vi "SystemdBControl.vi"(5 "Command":T1=enum."Connect dB", 6 "error in (no error)":errorcluster={"status"=TRUE, "code"=-2147467259, "source"="Exception occured in Microsoft OLE DB Provider for ODBC Drivers: no such table: sysconfig (1) in ADO Connection Execute.vi->SQL Execute.vi->dBManagerSQLite.vi->SystemdBControl.vi->ConfigSQLite.lvclass:ConfigGetLatestVersion.vi->SQLiteConfigOOP.vi->ConfigSQLiteOOP ini.vi\r\nSQL:Select Distinct\n  sysconfig.idsysconfig\nFrom\n  sysconfig\nOrder By\n  sysconfig.idsysconfig Desc\r\nSQL:Select\n  sysconfig.*\nFrom\n  sysconfig\nWhere\n  sysconfig.idsysconfig =   And\n  sysconfig.SectionName = \"\""}, 9 "Data In":variant) -> (0 "error out":errorcluster, 2 "Empty?":bool, 3 "Data Out":string[][](array[string]))   [LabVIEW 2023]
doc: "*-----------------------------------------------------\n* Author: SWatts\n*\n* VI Description: dB for all config stuff\n* \n*\n* Error handling: All errors passed out\n*\n* Pre-condition: \n*\n* Post-condition: None\n*\n* Revision History:\n*\n* Rev Date Author Description \n* 01 30/04/2014 SWatts First issue\n*\n*-----------------------------------------------------"
uses:
  SQLite/SQLiteLCOD.lvlib
  SQLite/SQLiteLCOD.ctl
  SystemdBCommands.ctl
panel:
  # "Input Data"
  # "Local Data"
  # "Output Data"
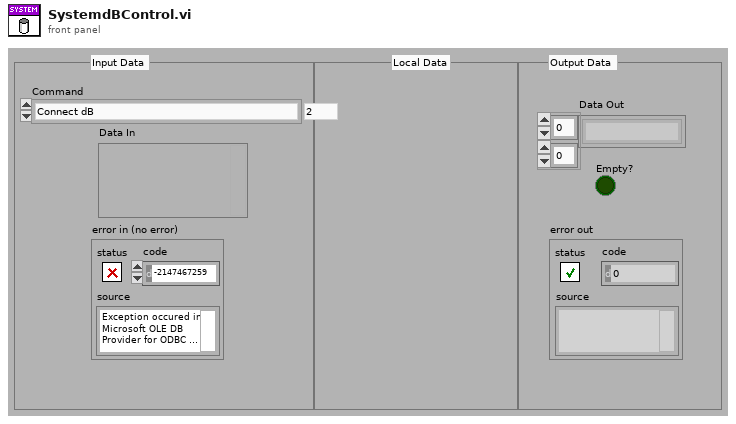
[diagram p1: front panel]
types:
  T1 = typedef "SystemdBCommands.ctl" = enum16{"No Command - Error", "Set Filepath", "Connect dB", "Disconnect dB", "Start Transaction", "Commit", "Rollback", "Describe Table", "Select All From Table", "Fetch Query", "Count Records In Table", "Get User Information", "Get System Config", "Insert New System Config", "UPDATE User Info", "Insert New User", "Get Versions", "Update Key", "Set Version to Default", "Get Default Version", "INSERT Error", "UPDATE Error", "DELETE Errors", "Get All Errors", "Get #Errors for Error"}
  T2 = typedef "SQLiteLCOD.lvlib/SQLiteLCOD.ctl" = enum16{"No Command - Error", "Open", "SQL", "Close", "Prepare SQL", "INSERT Waveform", "INSERT LongText", "Finalise SQL"}
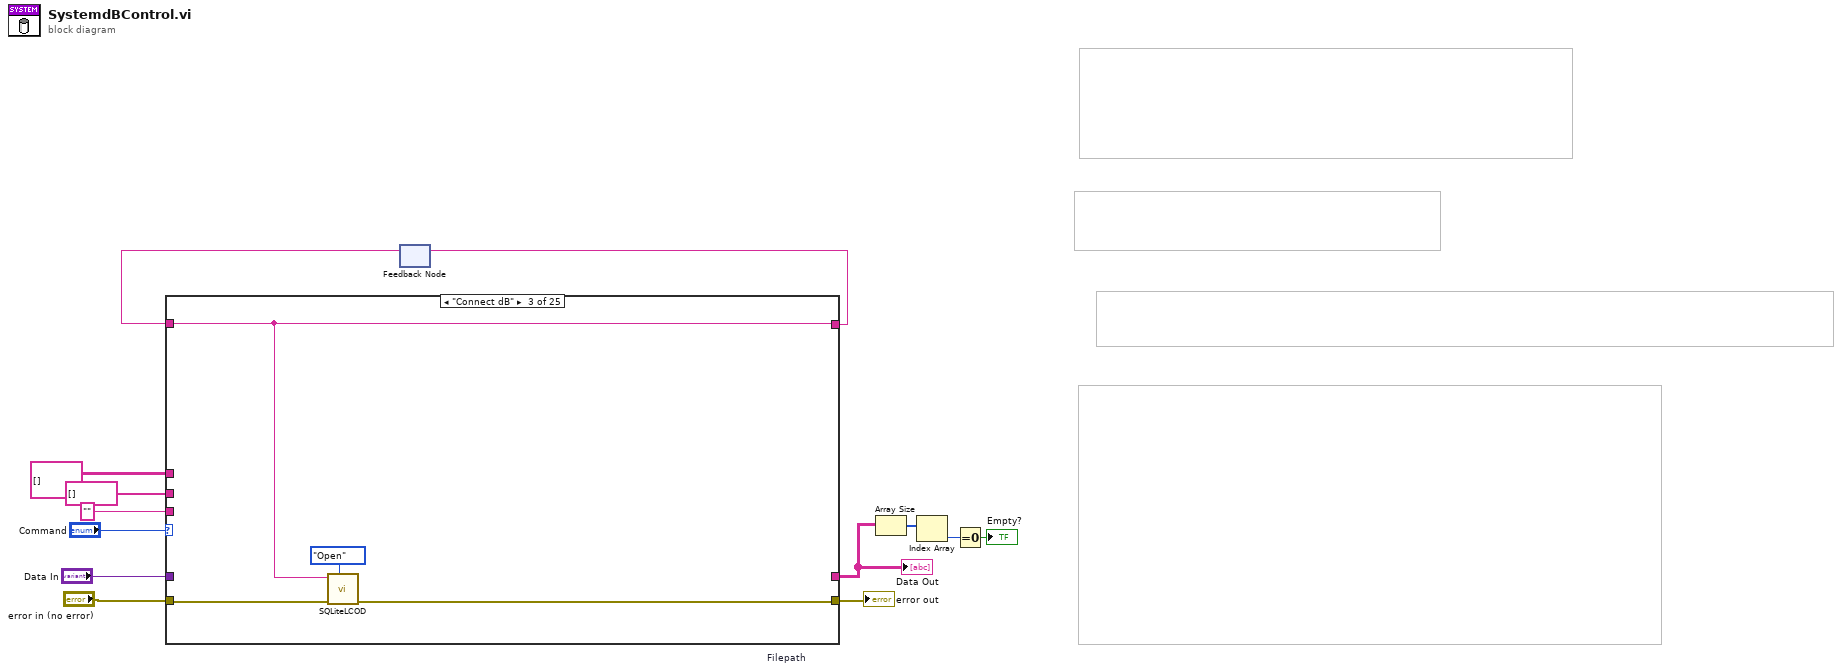
[diagram p0: block diagram]
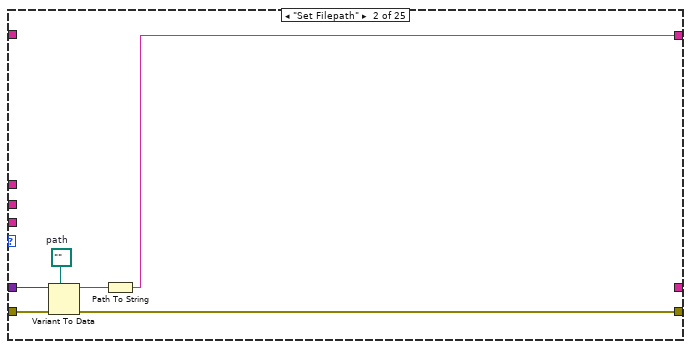
[diagram p3: hidden frame]
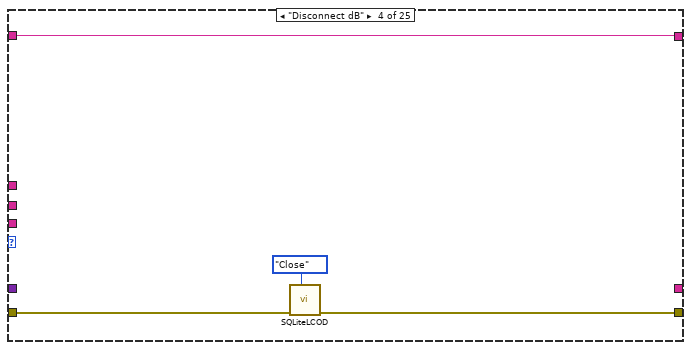
[diagram p4: hidden frame]
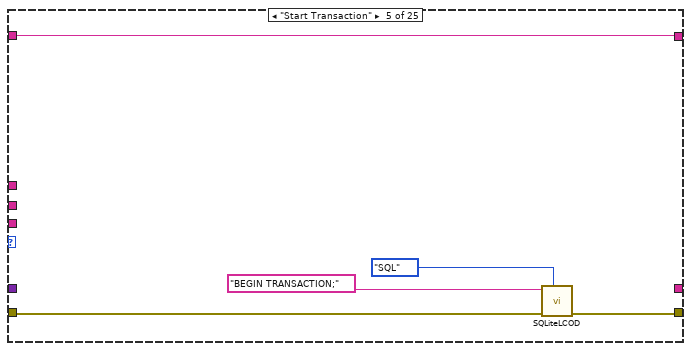
[diagram p5: hidden frame]
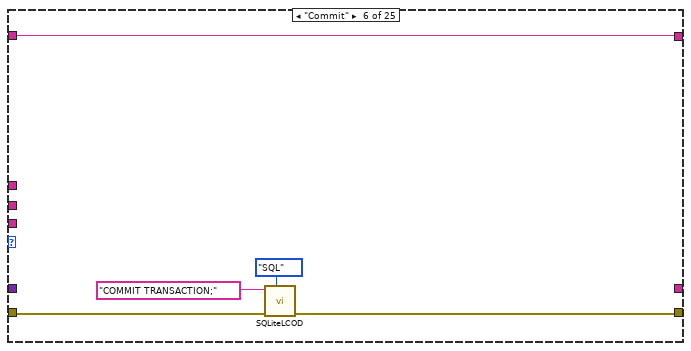
[diagram p6: hidden frame]
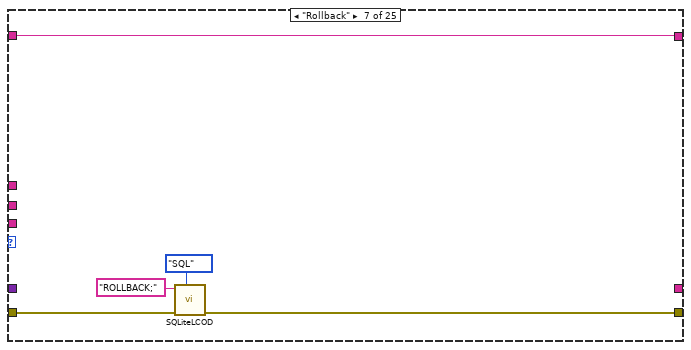
[diagram p7: hidden frame]
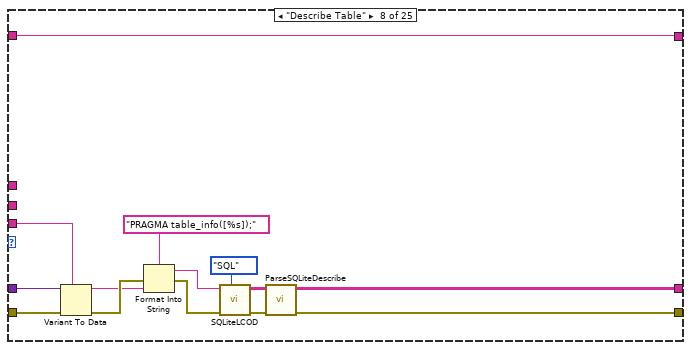
[diagram p8: hidden frame]
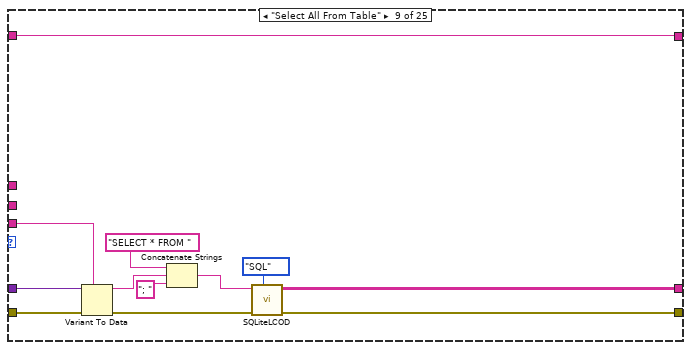
[diagram p9: hidden frame]
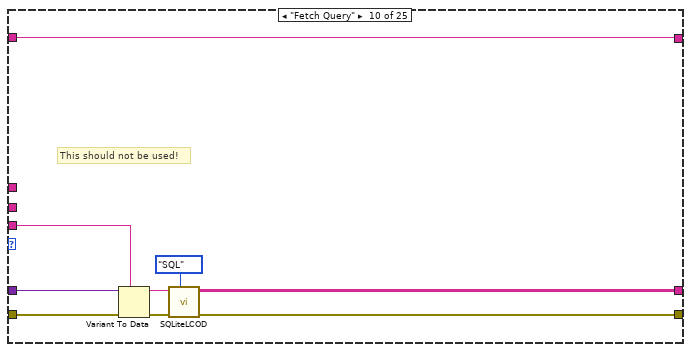
[diagram p10: hidden frame]
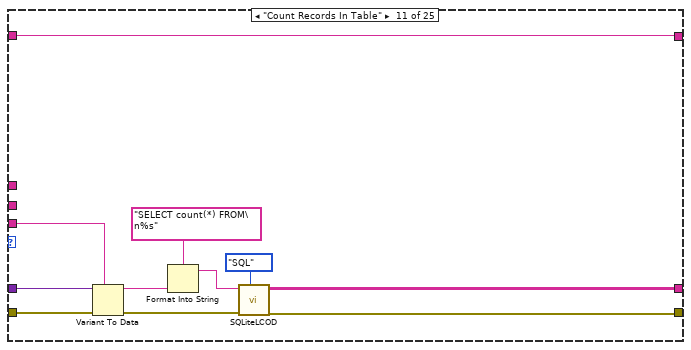
[diagram p11: hidden frame]
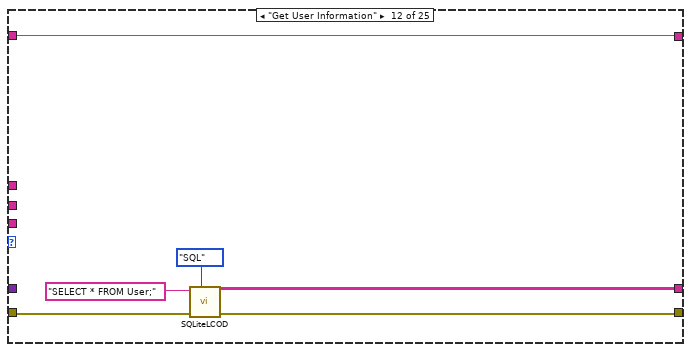
[diagram p12: hidden frame]
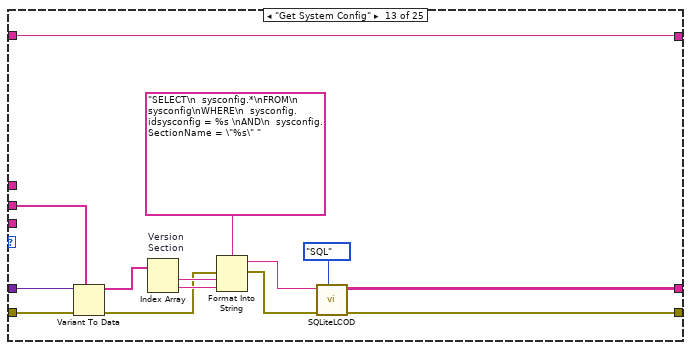
[diagram p13: hidden frame]
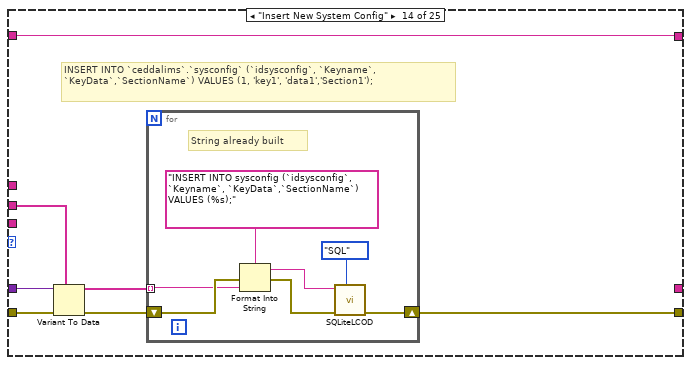
[diagram p14: hidden frame]
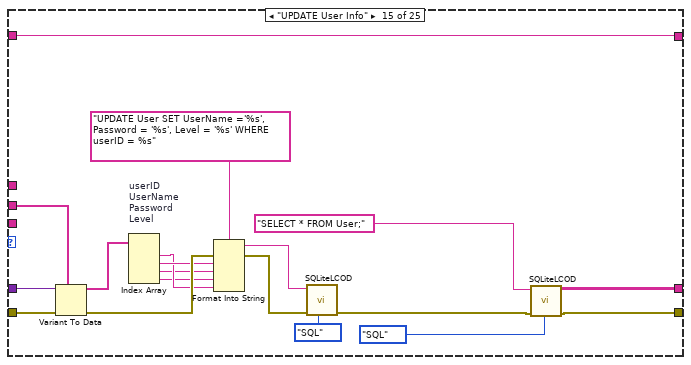
[diagram p15: hidden frame]
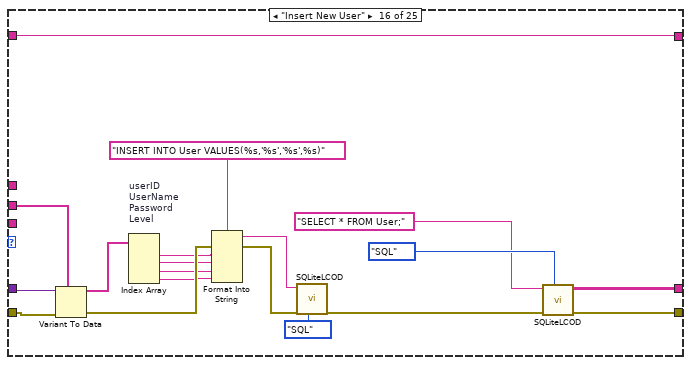
[diagram p16: hidden frame]
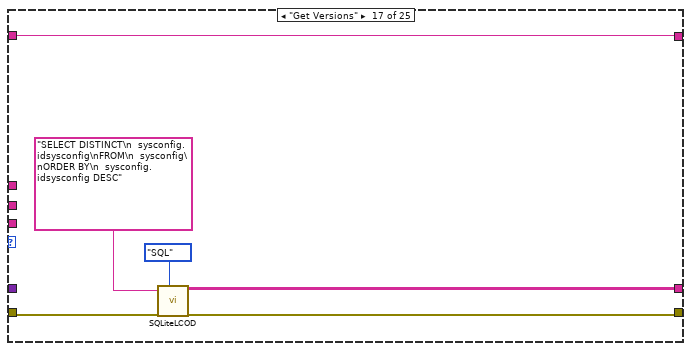
[diagram p17: hidden frame]
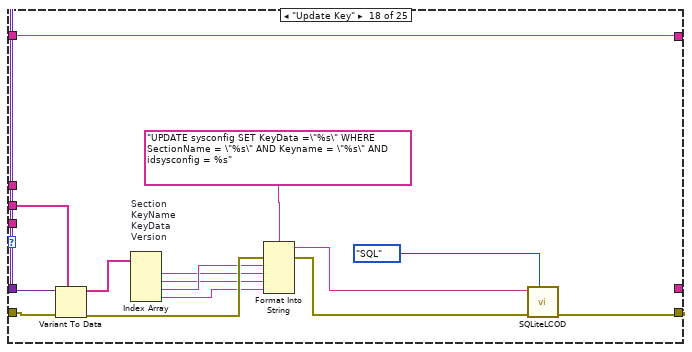
[diagram p18: hidden frame]
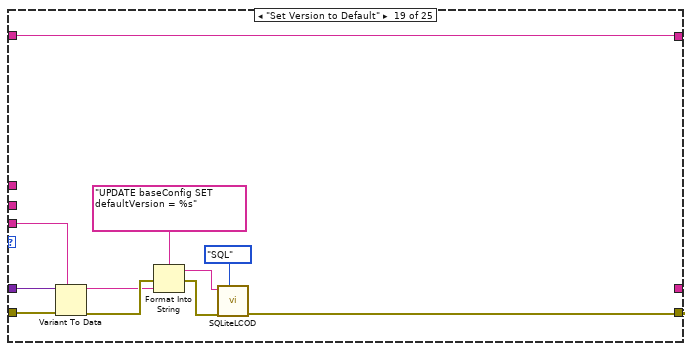
[diagram p19: hidden frame]
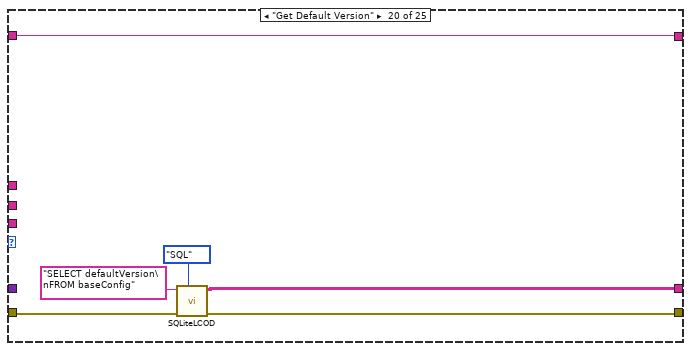
[diagram p20: hidden frame]
diagram:
  n1 = feedback #1 "Filepath"() -> (w1:string)  [unwired: 1 in]
  n2 = case shown="\"Connect dB\"" "Command" {
    tunnel: "error in (no error)" -> [w15 w20 w22 w28 w32 w38 w42 w56 w65 w78 w89 w94 w110 w117 w142 w161 w166 w182 w193 w198 w223 w237 w241 w247 w260]
    tunnel: "Data In" -> [_ w21 _ _ _ _ _ w57 w68 w79 w90 _ w109 w116 w141 w160 _ w181 w192 _ w222 w236 _ _ w259]
    tunnel: "" ("String") -> [_ _ _ _ _ _ _ w55 w66 w77 w88 _ _ _ _ _ _ _ w191 _ _ _ _ _ w258]
    tunnel: string[][] [] -> [_ _ _ _ _ _ _ _ _ _ _ _ _ _ _ _ _ _ _ _ _ _ _ _ _]
    tunnel: [w15 w18 w24 w27 w31 w36 w43 w54 w61 w72 w84 w95 w99 w112 w135 w156 w167 w177 w189 w199 w218 w232 w242 w248 w256] -> w12
    tunnel: string[] [] -> [_ _ _ _ _ _ _ _ _ _ _ _ w108 w115 w140 w159 _ w180 _ _ w221 w235 _ _ _]
    tunnel: [_ _ _ _ _ _ _ w53 w62 w73 w83 w93 w98 _ w136 w145 w164 _ _ w196 w210 _ w239 w245 w251] -> w5
    tunnel: [w14 w16 w23 w26 w30 w35 w40 w46 w59 w71 w80 w91 w97 w111 w125 w144 w163 w169 w185 w195 w209 w227 w238 w244 w252] -> w2
    tunnel: w1 -> [w14 _ w23 w26 w30 w35 w40 w46 w59 w71 w80 w91 w97 w111 w125 w144 w163 w169 w185 w195 w209 w227 w238 w244 w252]
    frame "No Command - Error", Default {
    }
    frame "Set Filepath" {
      w17 = path ""  # path
      n3 = Variant To Data(error in=w20, type=w17, Variant=w21) -> (data=w19:path, error out=w18:errorcluster)
      n4 = Path To String(path=w19) -> (string=w16:string)
    }
    frame "Connect dB" {
      n5 = call "SQLiteLCOD.vi"("dB Command"=SQLiteLCOD."Open", "error in (no error)"=w22, "String"=w23) -> ("error out"=w24:errorcluster)  [unwired: 4 in, 1 out]
    }
    frame "Disconnect dB" {
      n6 = call "SQLiteLCOD.vi"("dB Command"=SQLiteLCOD."Close", "error in (no error)"=w28) -> ("error out"=w27:errorcluster)  [unwired: 5 in, 1 out]
    }
    frame "Start Transaction" {
      n7 = call "SQLiteLCOD.vi"("dB Command"=SQLiteLCOD."SQL", "error in (no error)"=w32, "String"="BEGIN TRANSACTION;" ("Command Text")) -> ("error out"=w31:errorcluster)  [unwired: 4 in, 1 out]
    }
    frame "Commit" {
      n8 = call "SQLiteLCOD.vi"("dB Command"=SQLiteLCOD."SQL", "error in (no error)"=w38, "String"="COMMIT TRANSACTION;" ("Command Text")) -> ("error out"=w36:errorcluster)  [unwired: 4 in, 1 out]
    }
    frame "Rollback" {
      n9 = call "SQLiteLCOD.vi"("dB Command"=SQLiteLCOD."SQL", "error in (no error)"=w42, "String"="ROLLBACK;" ("Command Text")) -> ("error out"=w43:errorcluster)  [unwired: 4 in, 1 out]
    }
    frame "Describe Table" {
      n10 = Variant To Data(error in=w56, type=w55, Variant=w57) -> (data=w51:string, error out=w58:errorcluster)
      n11 = Format Into String(format string="PRAGMA table_info([%s]);", error in=w58, w51) -> (resulting string=w48:string, error out=w45:errorcluster)  [unwired: 1 in]
      n12 = call "SQLiteLCOD.vi"("dB Command"=SQLiteLCOD."SQL", "error in (no error)"=w45, "String"=w48) -> ("error out"=w49:errorcluster, "Rows"=w47:string[][])  [unwired: 4 in]
      n13 = call "ParseSQLiteDescribe.vi"("error in (no error)"=w49, "Data"=w47) -> ("error out"=w54:errorcluster, "appended array"=w53:string[][])  [unwired: 4 in]
    }
    frame "Select All From Table" {
      n14 = Variant To Data(error in=w65, type=w66, Variant=w68) -> (data=w67:string, error out=w60:errorcluster)
      n15 = Concatenate Strings("SELECT * FROM ", w67, "; ") -> (w63:string)
      n16 = call "SQLiteLCOD.vi"("dB Command"=SQLiteLCOD."SQL", "error in (no error)"=w60, "String"=w63) -> ("error out"=w61:errorcluster, "Rows"=w62:string[][])  [unwired: 4 in]
    }
    frame "Fetch Query" {
      # "This should not be used!"
      n17 = Variant To Data(error in=w78, type=w77, Variant=w79) -> (data=w74:string, error out=w75:errorcluster)
      n18 = call "SQLiteLCOD.vi"("dB Command"=SQLiteLCOD."SQL", "error in (no error)"=w75, "String"=w74) -> ("error out"=w72:errorcluster, "Rows"=w73:string[][])  [unwired: 4 in]
    }
    frame "Count Records In Table" {
      n19 = Variant To Data(error in=w89, type=w88, Variant=w90) -> (data=w86:string, error out=w82:errorcluster)
      n20 = Format Into String(format string="SELECT count(*) FROM\n%s", w86) -> (resulting string=w81:string)  [unwired: 2 in, 1 out]
      n21 = call "SQLiteLCOD.vi"("dB Command"=SQLiteLCOD."SQL", "error in (no error)"=w82, "String"=w81) -> ("error out"=w84:errorcluster, "Rows"=w83:string[][])  [unwired: 4 in]
    }
    frame "Get User Information" {
      n22 = call "SQLiteLCOD.vi"("dB Command"=SQLiteLCOD."SQL", "error in (no error)"=w94, "String"="SELECT * FROM User;") -> ("error out"=w95:errorcluster, "Rows"=w93:string[][])  [unwired: 4 in]
    }
    frame "Get System Config" {
      n23 = Variant To Data(error in=w110, type=w108, Variant=w109) -> (data=w107:string[], error out=w103:errorcluster)
      n24 = Index Array "Version\nSection"(array=w107) -> (element #1=w105:string, element #2=w104:string)  [unwired: 2 in]
      n25 = Format Into String(format string="SELECT\n  sysconfig.*\nFROM\n  sysconfig\nWHERE\n  sysconfig.idsysconfig = %s \nAND\n  sysconfig.SectionName = \"%s\" " ("String"), error in=w103, w105, w104) -> (resulting string=w100:string, error out=w101:errorcluster)  [unwired: 1 in]
      n26 = call "SQLiteLCOD.vi"("dB Command"=SQLiteLCOD."SQL", "error in (no error)"=w101, "String"=w100) -> ("error out"=w99:errorcluster, "Rows"=w98:string[][])  [unwired: 4 in]
    }
    frame "Insert New System Config" {
      # "INSERT INTO `ceddalims`.`sysconfig` (`idsysconfig`, `Keyname`, `KeyData`,`SectionName`) VALUES (1, 'key1', 'data1','Section1');"
      n27 = Variant To Data(error in=w117, type=w115, Variant=w116) -> (data=w114:string[], error out=w113:errorcluster)
      n28 = for {
        tunnel: w114 -> [w122] mode=indexing
        shift-right: [w120] -> w112
        shift-left: w113 -> [w124]
        # "String already built"
        n29 = Format Into String(format string="INSERT INTO sysconfig (`idsysconfig`, `Keyname`, `KeyData`,`SectionName`) VALUES (%s);" ("String"), error in=w124, w122) -> (resulting string=w119:string, error out=w118:errorcluster)  [unwired: 1 in]
        n30 = call "SQLiteLCOD.vi"("dB Command"=SQLiteLCOD."SQL", "error in (no error)"=w118, "String"=w119) -> ("error out"=w120:errorcluster)  [unwired: 4 in, 1 out]
      }
    }
    frame "UPDATE User Info" {
      n31 = Variant To Data(error in=w142, type=w140, Variant=w141) -> (data=w139:string[], error out=w143:errorcluster)
      n32 = Index Array "userID\nUserName\nPassword\nLevel"(array=w139) -> (element #1=w130:string, element #2=w131:string, element #3=w129:string, element #4=w128:string)  [unwired: 4 in]
      n33 = Format Into String(format string="UPDATE User SET UserName ='%s', Password = '%s', Level = '%s' WHERE userID = %s" ("String"), error in=w143, w131, w129, w128, w130) -> (resulting string=w126:string, error out=w127:errorcluster)  [unwired: 1 in]
      n34 = call "SQLiteLCOD.vi"("dB Command"=SQLiteLCOD."SQL", "error in (no error)"=w127, "String"=w126) -> ("error out"=w137:errorcluster)  [unwired: 4 in, 1 out]
      n35 = call "SQLiteLCOD.vi"("dB Command"=SQLiteLCOD."SQL", "error in (no error)"=w137, "String"="SELECT * FROM User;") -> ("error out"=w135:errorcluster, "Rows"=w136:string[][])  [unwired: 4 in]
    }
    frame "Insert New User" {
      n36 = Variant To Data(error in=w161, type=w159, Variant=w160) -> (data=w158:string[], error out=w162:errorcluster)
      n37 = Index Array "userID\nUserName\nPassword\nLevel"(array=w158) -> (element #1=w151:string, element #2=w150:string, element #3=w149:string, element #4=w148:string)  [unwired: 4 in]
      n38 = Format Into String(format string="INSERT INTO User VALUES(%s,'%s','%s',%s)" ("String"), error in=w162, w151, w150, w149, w148) -> (resulting string=w147:string, error out=w146:errorcluster)  [unwired: 1 in]
      n39 = call "SQLiteLCOD.vi"("dB Command"=SQLiteLCOD."SQL", "error in (no error)"=w146, "String"=w147) -> ("error out"=w154:errorcluster)  [unwired: 4 in, 1 out]
      n40 = call "SQLiteLCOD.vi"("dB Command"=SQLiteLCOD."SQL", "error in (no error)"=w154, "String"="SELECT * FROM User;") -> ("error out"=w156:errorcluster, "Rows"=w145:string[][])  [unwired: 4 in]
    }
    frame "Get Versions" {
      n41 = call "SQLiteLCOD.vi"("dB Command"=SQLiteLCOD."SQL", "error in (no error)"=w166, "String"="SELECT DISTINCT\n  sysconfig.idsysconfig\nFROM\n  sysconfig\nORDER BY\n  sysconfig.idsysconfig DESC") -> ("error out"=w167:errorcluster, "Rows"=w164:string[][])  [unwired: 4 in]
    }
    frame "Update Key" {
      n42 = Variant To Data(error in=w182, type=w180, Variant=w181) -> (data=w179:string[], error out=w183:errorcluster)
      n43 = Index Array "Section\nKeyName\nKeyData\nVersion"(array=w179) -> (element #1=w174:string, element #2=w173:string, element #3=w175:string, element #4=w172:string)  [unwired: 4 in]
      n44 = Format Into String(format string="UPDATE sysconfig SET KeyData =\"%s\" WHERE SectionName = \"%s\" AND Keyname = \"%s\" AND idsysconfig = %s" ("String"), error in=w183, w175, w174, w173, w172) -> (resulting string=w171:string, error out=w170:errorcluster)  [unwired: 1 in]
      n45 = call "SQLiteLCOD.vi"("dB Command"=SQLiteLCOD."SQL", "error in (no error)"=w170, "String"=w171) -> ("error out"=w177:errorcluster)  [unwired: 4 in, 1 out]
    }
    frame "Set Version to Default" {
      n46 = Variant To Data(error in=w193, type=w191, Variant=w192) -> (data=w187:string, error out=w194:errorcluster)
      n47 = Format Into String(format string="UPDATE baseConfig SET defaultVersion = %s" ("String"), error in=w194, w187) -> (resulting string=w186:string, error out=w184:errorcluster)  [unwired: 1 in]
      n48 = call "SQLiteLCOD.vi"("dB Command"=SQLiteLCOD."SQL", "error in (no error)"=w184, "String"=w186) -> ("error out"=w189:errorcluster)  [unwired: 4 in, 1 out]
    }
    frame "Get Default Version" {
      n49 = call "SQLiteLCOD.vi"("dB Command"=SQLiteLCOD."SQL", "error in (no error)"=w198, "String"="SELECT defaultVersion\nFROM baseConfig") -> ("error out"=w199:errorcluster, "Rows"=w196:string[][])  [unwired: 4 in]
    }
    frame "INSERT Error" {
      w204 = "?"  # Bind Column
      n50 = Variant To Data(error in=w223, type=w221, Variant=w222) -> (data=w220:string[], error out=w224:errorcluster)
      n51 = Index Array "errorNumber\nerrorSource\ntotalErrors\nlastErrorDate"(array=w220) -> (element #1=w215:string, element #2=w205:string, element #3=w214:string, element #4=w213:string)  [unwired: 4 in]
      n52 = Format Into String(format string="INSERT INTO errorlog (\"errorNumber\", \"errorSource\", \"totalErrors\", \"lastErrorDate\") VALUES (%s, %s, %s, '%s')" ("String"), error in=w224, w215, w204, w214, w213) -> (resulting string=w212:string, error out=w211:errorcluster)  [unwired: 1 in]
      n53 = call "SQLiteLCOD.vi"("dB Command"=SQLiteLCOD."Prepare SQL", "error in (no error)"=w211, "String"=w212) -> ("error out"=w207:errorcluster)  [unwired: 4 in, 1 out]
      n54 = call "SQLiteLCOD.vi"("dB Command"=SQLiteLCOD."INSERT LongText", "error in (no error)"=w207, "String"=w205) -> ("error out"=w203:errorcluster)  [unwired: 4 in, 1 out]
      n55 = call "SQLiteLCOD.vi"("dB Command"=SQLiteLCOD."Finalise SQL", "error in (no error)"=w203) -> ("error out"=w202:errorcluster)  [unwired: 5 in, 1 out]
      n56 = call "SQLiteLCOD.vi"("dB Command"=SQLiteLCOD."SQL", "error in (no error)"=w202, "String"="SELECT * FROM errorlog") -> ("error out"=w218:errorcluster, "Rows"=w210:string[][])  [unwired: 4 in]
    }
    frame "UPDATE Error" {
      n57 = Variant To Data(error in=w237, type=w235, Variant=w236) -> (data=w234:string[], error out=w230:errorcluster)
      n58 = Index Array "ErrorNumber\nnumErrors"(array=w234) -> (element #1=w225:string, element #2=w226:string)  [unwired: 2 in]
      n59 = Format Into String(format string="UPDATE errorlog SET \"totalErrors\"=%s WHERE (\"errorNumber\"=%s)" ("String"), error in=w230, w226, w225) -> (resulting string=w229:string, error out=w228:errorcluster)  [unwired: 1 in]
      n60 = call "SQLiteLCOD.vi"("dB Command"=SQLiteLCOD."SQL", "error in (no error)"=w228, "String"=w229) -> ("error out"=w232:errorcluster)  [unwired: 4 in, 1 out]
    }
    frame "DELETE Errors" {
      n61 = call "SQLiteLCOD.vi"("dB Command"=SQLiteLCOD."SQL", "error in (no error)"=w241, "String"="DELETE FROM errorlog") -> ("error out"=w242:errorcluster, "Rows"=w239:string[][])  [unwired: 4 in]
    }
    frame "Get All Errors" {
      n62 = call "SQLiteLCOD.vi"("dB Command"=SQLiteLCOD."SQL", "error in (no error)"=w247, "String"="SELECT * FROM errorlog") -> ("error out"=w248:errorcluster, "Rows"=w245:string[][])  [unwired: 4 in]
    }
    frame "Get #Errors for Error" {
      n63 = Variant To Data(error in=w260, type=w258, Variant=w259) -> (data=w254:string, error out=w261:errorcluster)
      n64 = Format Into String(format string="SELECT\nerrorlog.totalErrors\nFROM\nerrorlog\nWHERE\nerrorlog.errorNumber = %s" ("String"), error in=w261, w254) -> (resulting string=w253:string, error out=w250:errorcluster)  [unwired: 1 in]
      n65 = call "SQLiteLCOD.vi"("dB Command"=SQLiteLCOD."SQL", "error in (no error)"=w250, "String"=w253) -> ("error out"=w256:errorcluster, "Rows"=w251:string[][])  [unwired: 4 in]
    }
  }
  "error out" <- w12
  "Data Out" <- w5
  n66 = feedback-in #1(w2) -> ()
  n67 = Array Size(array=w5) -> (size(s)=w4:i32[])
  n68 = Index Array(array=w4) -> (element=w3:i32)  [unwired: 1 in]
  n69 = Equal To 0?(x=w3) -> (x = 0?=→"Empty?":bool)
